vi "WaveformVisualiserLab10.vi"() -> ()   [LabVIEW 2021]
uses:
  <vilib>/Instr/_visa.llb/VISA Flush IO Buffer Mask.ctl
  <vilib>/Analysis/baseanly.llb/Mean (DBL).vi
  <vilib>/Instr/_visa.llb/VISA Configure Serial Port (Instr).vi
  <vilib>/measure/maspectr.llb/FFT Spectrum (Mag-Phase) for 1 Chan.vi
  <vilib>/measure/NI_MAPro.lvlib
  <vilib>/Analysis/NI_AALBase.lvlib
panel:
  out "Waveform Graph":cluster{"f0":dbl, "df":dbl, "magnitude":dbl[]}(graph)
  out "XY Graph 2":cluster{i32[], dbl[]}[](graph)
  out "error out":errorcluster
  in  "write buffer":string
  # "Remember to change your com port to match the port used by your IBM4"
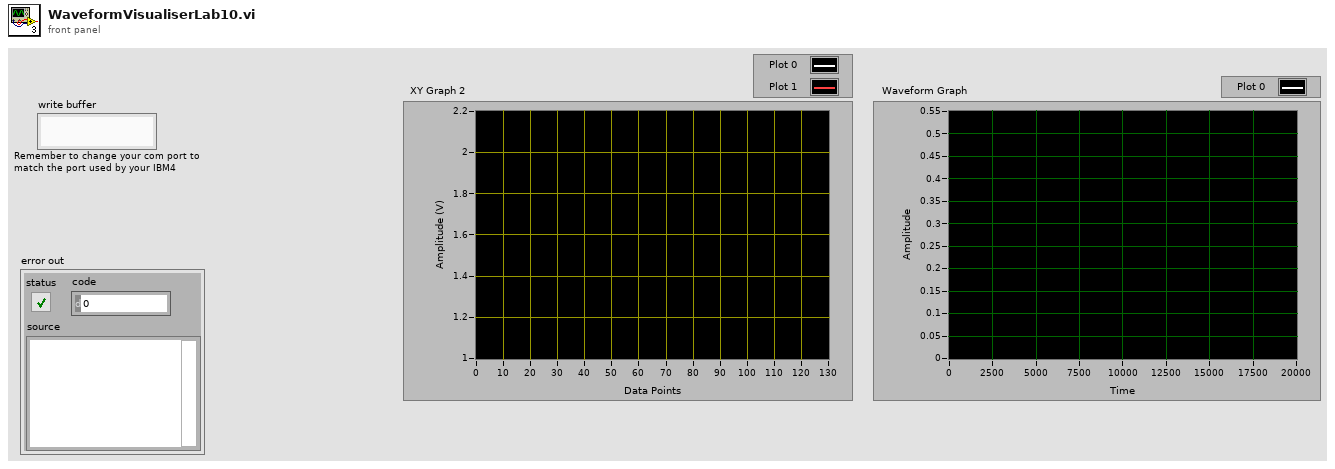
[diagram p1: front panel]
types:
  T1 = typedef "VISA Flush IO Buffer Mask.ctl" = u16
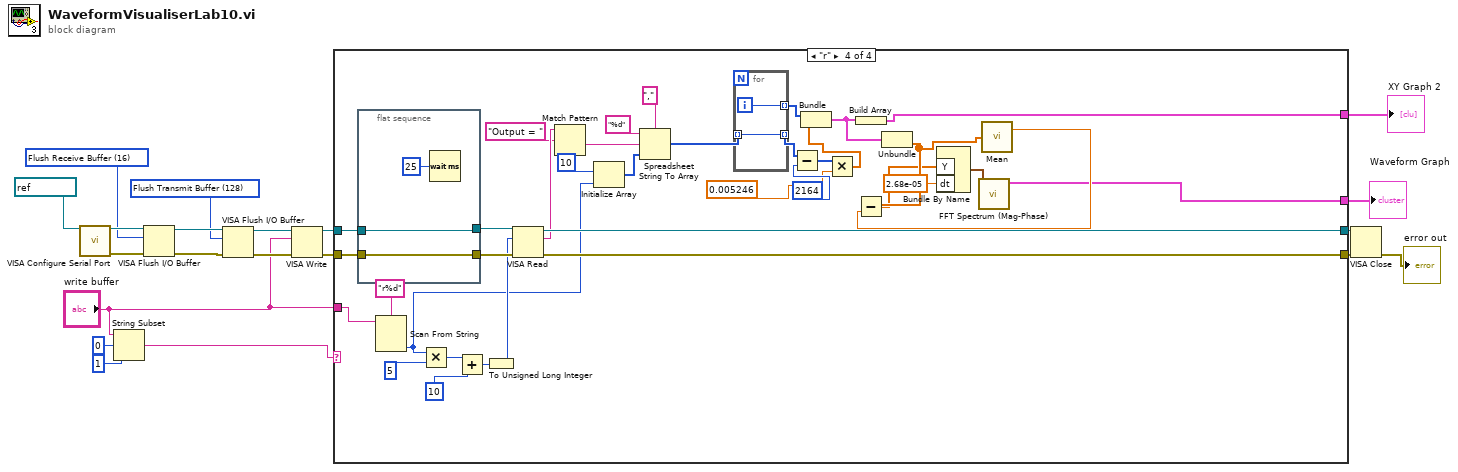
[diagram p0: block diagram]
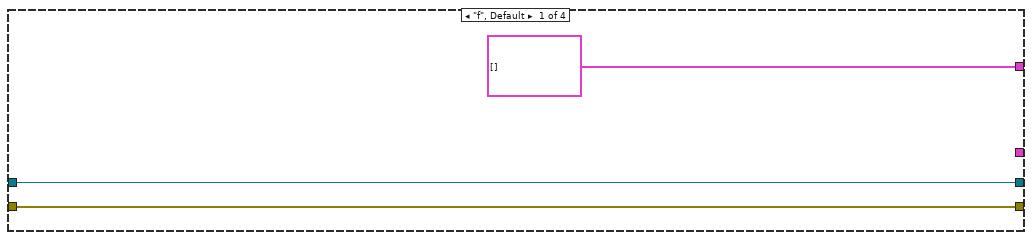
[diagram p2: hidden frame]
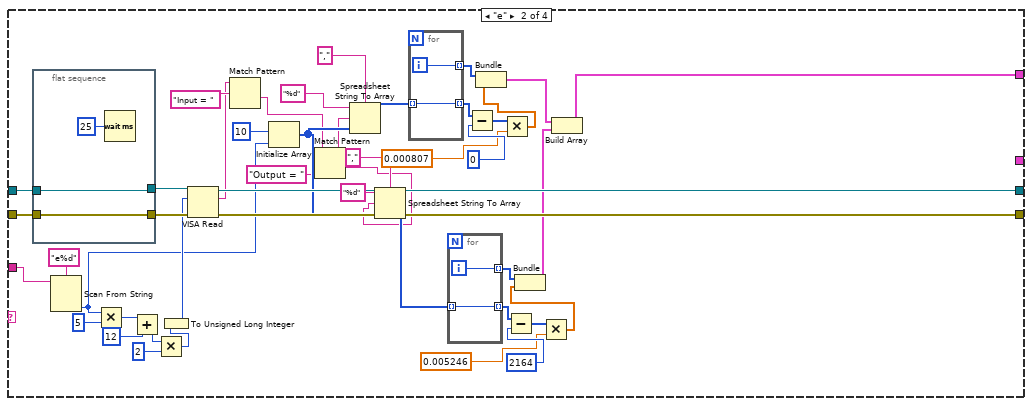
[diagram p3: hidden frame]
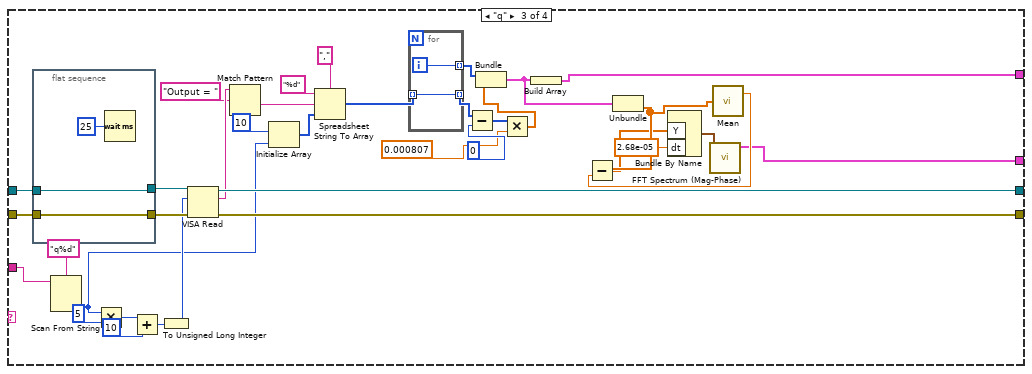
[diagram p4: hidden frame]
diagram:
  w14 = T1 128 items=["Flush Receive Buffer"=16, "Write Transmit Buffer to Device"=32, "Flush Receive Buffer (No I/O)"=64, "Flush Transmit Buffer"=128] ("Mask")
  w17 = T1 16 items=["Flush Receive Buffer"=16, "Write Transmit Buffer to Device"=32, "Flush Receive Buffer (No I/O)"=64, "Flush Transmit Buffer"=128] ("Mask")
  n1 = call-poly "VISA Configure Serial Port"("VISA resource name"=refnum<visa-resource-name> "COM5") -> ("VISA resource name out"=w19:refnum<visa-resource-name>, "error out"=w18:errorcluster)  [unwired: 13 in]
  n2 = String Subset(string="write buffer", offset (0)=0, length (rest)=1 ("length (rest)")) -> (substring=w3:string)
  n3 = VISA Flush I/O Buffer(VISA resource name=w19, mask (16)=w17, error in (no error)=w18) -> (VISA resource name out=w16:refnum<visa-resource-name>, error out=w15:errorcluster)
  n4 = VISA Flush I/O Buffer(VISA resource name=w16, mask (16)=w14, error in (no error)=w15) -> (VISA resource name out=w13:refnum<visa-resource-name>, error out=w12:errorcluster)
  n5 = VISA Write(VISA resource name=w13, write buffer="write buffer", error in (no error)=w12) -> (VISA resource name out=w8:refnum<visa-resource-name>, error out=w7:errorcluster)  [unwired: 1 out]
  n6 = case shown="\"r\"" w3 {
    tunnel: [w22 w68 w111 w152] -> w11
    tunnel: [w23 w67 w110 w151] -> w10
    tunnel: w8 -> [w23 w66 w109 w150]
    tunnel: w7 -> [w22 w64 w107 w148]
    tunnel: "write buffer" -> [_ w62 w105 w146]
    tunnel: [cluster{i32[], dbl[]}[] [] w31 w83 w124] -> w2
    tunnel: [_ _ w76 w117] -> w1
    frame "f", Default {
    }
    frame "e" {
      n7 = flat-sequence {
        tunnel: [w75] -> w65
        tunnel: w66 -> [w75]
        tunnel: [w74] -> w63
        tunnel: w64 -> [w74]
        frame #0 {
          n8 = Wait (ms)(milliseconds to wait=u32 25) -> ()  [unwired: 1 out]
        }
      }
      n9 = Scan From String(format string="e%d", input string=w62) -> (output 1=w52:i32)  [unwired: 3 in, 3 out]
      n10 = Multiply(x=w52, y=5) -> (x*y=w59:i32)
      n11 = Add(x=w59, y=12) -> (x+y=w44:i32)
      n12 = Multiply(x=w44, y=2) -> (x*y=w27:i32)
      n13 = To Unsigned Long Integer(number=w27) -> (unsigned 32bit integer=w57:u32)
      n14 = VISA Read(VISA resource name=w65, byte count=w57, error in (no error)=w63) -> (VISA resource name out=w67:refnum<visa-resource-name>, read buffer=w26:string, error out=w68:errorcluster)  [unwired: 1 out]
      n15 = Match Pattern(string=w26, regular expression="Input = ") -> (after substring=w25:string)  [unwired: 1 in, 3 out]
      n16 = Initialize Array(10 ("y"), w52) -> (w42:i32[])
      n17 = Match Pattern(string=w25, regular expression="Output = ") -> (before substring=w24:string, after substring=w28:string)  [unwired: 1 in, 2 out]
      n18 = Spreadsheet String To Array(delimiter (Tab)=",", format string="%d", spreadsheet string=w24, array type (2D Dbl)=w42) -> (array=w51:i32[])
      n19 = Spreadsheet String To Array(delimiter (Tab)=",", format string="%d", spreadsheet string=w28, array type (2D Dbl)=w42) -> (array=w36:i32[])
      n20 = for {
        tunnel: w51 -> [w72] mode=indexing
        tunnel: [w72] -> w48 mode=indexing
        tunnel: [w71] -> w50 mode=indexing
        i -> [w71]
      }
      n21 = for {
        tunnel: w36 -> [w70] mode=indexing
        tunnel: [w70] -> w39 mode=indexing
        tunnel: [w69] -> w41 mode=indexing
        i -> [w69]
      }
      n22 = Subtract(x=w48, y=0) -> (x-y=w47:i32[])
      n23 = Multiply(x=w47, y=0.000807) -> (x*y=w45:dbl[])
      n24 = Bundle(w50, w45) -> (w33:cluster{i32[], dbl[]})  [unwired: 1 in]
      n25 = Subtract(x=w39, y=2164) -> (x-y=w38:i32[])
      n26 = Multiply(x=w38, y=0.005246) -> (x*y=w34:dbl[])
      n27 = Bundle(w41, w34) -> (w32:cluster{i32[], dbl[]})  [unwired: 1 in]
      n28 = Build Array(w33, w32) -> (w31:cluster{i32[], dbl[]}[])
    }
    frame "q" {
      n29 = flat-sequence {
        tunnel: [w116] -> w108
        tunnel: w109 -> [w116]
        tunnel: [w115] -> w106
        tunnel: w107 -> [w115]
        frame #0 {
          n30 = Wait (ms)(milliseconds to wait=u32 25) -> ()  [unwired: 1 out]
        }
      }
      n31 = Scan From String(format string="q%d", input string=w105) -> (output 1=w92:i32)  [unwired: 3 in, 3 out]
      n32 = Multiply(x=w92, y=5) -> (x*y=w102:i32)
      n33 = Add(x=w102, y=10) -> (x+y=w100:i32)
      n34 = To Unsigned Long Integer(number=w100) -> (unsigned 32bit integer=w99:u32)
      n35 = VISA Read(VISA resource name=w108, byte count=w99, error in (no error)=w106) -> (VISA resource name out=w110:refnum<visa-resource-name>, read buffer=w98:string, error out=w111:errorcluster)  [unwired: 1 out]
      n36 = Match Pattern(string=w98, regular expression="Output = ") -> (after substring=w96:string)  [unwired: 1 in, 3 out]
      n37 = Initialize Array(10 ("y"), w92) -> (w91:i32[])
      n38 = Spreadsheet String To Array(delimiter (Tab)=",", format string="%d", spreadsheet string=w96, array type (2D Dbl)=w91) -> (array=w90:i32[])
      n39 = for {
        tunnel: w90 -> [w113] mode=indexing
        tunnel: [w113] -> w87 mode=indexing
        tunnel: [w112] -> w89 mode=indexing
        i -> [w112]
      }
      n40 = Subtract(x=w87, y=0) -> (x-y=w86:i32[])
      n41 = Multiply(x=w86, y=0.000807) -> (x*y=w84:dbl[])
      n42 = Bundle(w89, w84) -> (w78:cluster{i32[], dbl[]})  [unwired: 1 in]
      n43 = Build Array(w78) -> (w83:cluster{i32[], dbl[]}[])
      n44 = Unbundle(w78) -> (w80:dbl[])  [unwired: 1 out]
      n45 = call-poly <vilib>:"Mean.vi"("X"=w80) -> ("mean"=w77:dbl)  [unwired: 1 out]
      n46 = Subtract(x=w80, y=w77) -> (x-y=w79:dbl[])
      n47 = Bundle By Name("Y"=w79, "dt"=2.68e-05) -> (w81:waveform(dbl))  [unwired: 1 in]
      n48 = call-poly <vilib>:"FFT Spectrum (Mag-Phase).vi"("time signal"=w81) -> ("magnitude"=w76:cluster{"f0":dbl, "df":dbl, "magnitude":dbl[]})  [unwired: 6 in, 4 out]
    }
    frame "r" {
      n49 = flat-sequence {
        tunnel: [w157] -> w149
        tunnel: w150 -> [w157]
        tunnel: [w156] -> w147
        tunnel: w148 -> [w156]
        frame #0 {
          n50 = Wait (ms)(milliseconds to wait=u32 25) -> ()  [unwired: 1 out]
        }
      }
      n51 = Scan From String(format string="r%d", input string=w146) -> (output 1=w133:i32)  [unwired: 3 in, 3 out]
      n52 = Multiply(x=w133, y=5) -> (x*y=w143:i32)
      n53 = Add(x=w143, y=10) -> (x+y=w141:i32)
      n54 = To Unsigned Long Integer(number=w141) -> (unsigned 32bit integer=w140:u32)
      n55 = VISA Read(VISA resource name=w149, byte count=w140, error in (no error)=w147) -> (VISA resource name out=w151:refnum<visa-resource-name>, read buffer=w139:string, error out=w152:errorcluster)  [unwired: 1 out]
      n56 = Match Pattern(string=w139, regular expression="Output = ") -> (after substring=w137:string)  [unwired: 1 in, 3 out]
      n57 = Initialize Array(10 ("y"), w133) -> (w132:i32[])
      n58 = Spreadsheet String To Array(delimiter (Tab)=",", format string="%d", spreadsheet string=w137, array type (2D Dbl)=w132) -> (array=w131:i32[])
      n59 = for {
        tunnel: w131 -> [w154] mode=indexing
        tunnel: [w154] -> w128 mode=indexing
        tunnel: [w153] -> w130 mode=indexing
        i -> [w153]
      }
      n60 = Subtract(x=w128, y=2164) -> (x-y=w127:i32[])
      n61 = Multiply(x=w127, y=0.005246) -> (x*y=w125:dbl[])
      n62 = Bundle(w130, w125) -> (w123:cluster{i32[], dbl[]})  [unwired: 1 in]
      n63 = Build Array(w123) -> (w124:cluster{i32[], dbl[]}[])
      n64 = Unbundle(w123) -> (w120:dbl[])  [unwired: 1 out]
      n65 = call-poly <vilib>:"Mean.vi"("X"=w120) -> ("mean"=w119:dbl)  [unwired: 1 out]
      n66 = Subtract(x=w120, y=w119) -> (x-y=w118:dbl[])
      n67 = Bundle By Name("Y"=w118, "dt"=2.68e-05) -> (w121:waveform(dbl))  [unwired: 1 in]
      n68 = call-poly <vilib>:"FFT Spectrum (Mag-Phase).vi"("time signal"=w121) -> ("magnitude"=w117:cluster{"f0":dbl, "df":dbl, "magnitude":dbl[]})  [unwired: 6 in, 4 out]
    }
  }
  "XY Graph 2" <- w2
  "Waveform Graph" <- w1
  n69 = VISA Close(VISA resource name=w10, error in (no error)=w11) -> (error out=→"error out":errorcluster)
